vi "Format timestamp into string vs Get Time String.vi"() -> ()   [LabVIEW 2020]
panel:
  out "concatenated string 2":string
  out "concatenated string":string
  out "unit (ms) 2":dbl[](graph)
  out "inside 2":i32
  out "outside 2":i32
  out "inside":i32
  out "outside":i32
  out "unit (ms)":dbl[][](graph)
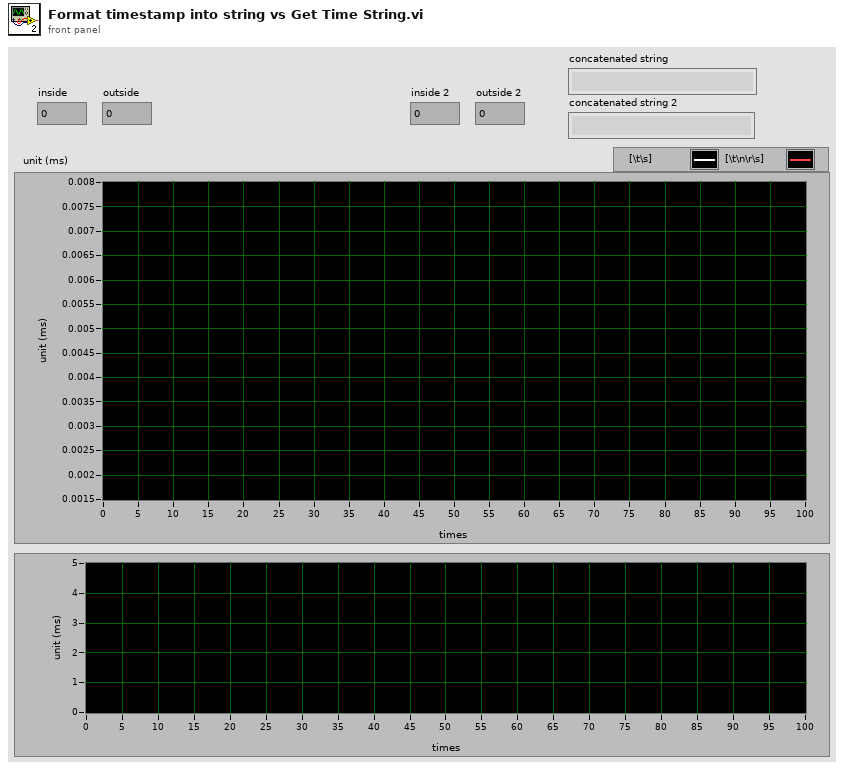
[diagram p1: front panel]
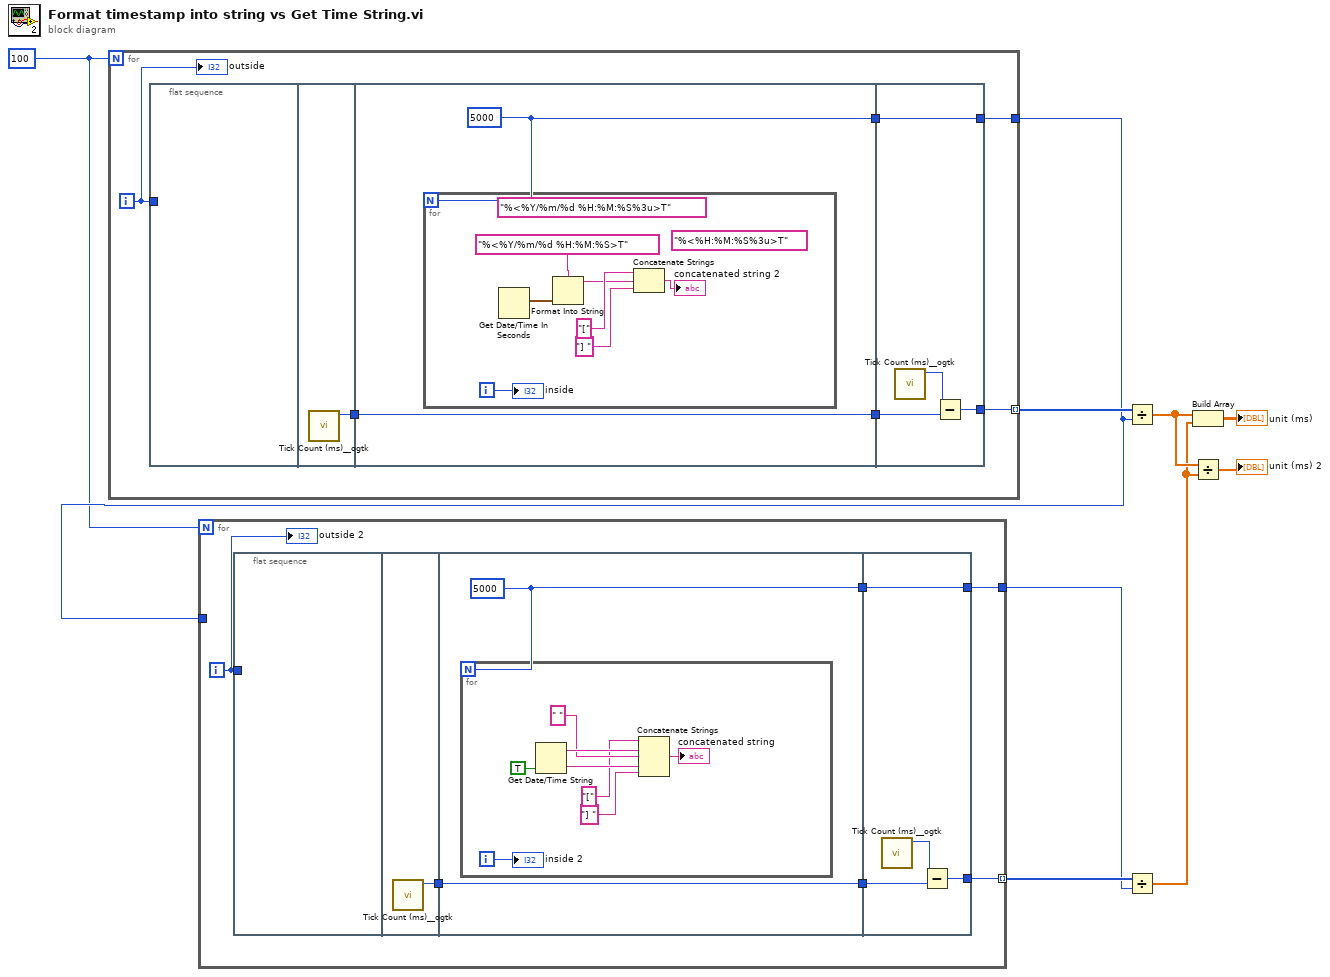
[diagram p0: block diagram]
diagram:
  w4 = 100
  n1 = for {
    N: w4 -> [_]
    tunnel: [w13] -> w9 mode=indexing
    tunnel: [w12] -> w5
    i -> [w10]
    n2 = flat-sequence {
      tunnel: w10 -> [_]
      tunnel: [w16] -> w15
      tunnel: w15 -> [w18]
      tunnel: [w18] -> w14
      tunnel: [w17] -> w11
      tunnel: w14 -> [w28]
      tunnel: [w27] -> w13
      tunnel: [w26] -> w12
      tunnel: w11 -> [w26]
      frame #0 {
      }
      frame #1 {
        n3 = call <userlib>:"Tick Count (ms)__ogtk.vi"() -> ("millisecond timer value"=w16:u32)  [unwired: 10 in, 1 out]
      }
      frame #2 {
        w17 = 5000
        n4 = for {
          N: w17 -> [_]
          i -> [w25]
          (unwired) "%<%H:%M:%S%3u>T" ("format string")
          (unwired) "%<%Y/%m/%d %H:%M:%S%3u>T" ("format string")
          n5 = Get Date/Time In Seconds() -> (seconds since 1Jan1904=w22:timestamp)
          n6 = Format Into String(format string="%<%Y/%m/%d %H:%M:%S>T", w22) -> (resulting string=w21:string)  [unwired: 2 in, 1 out]
          n7 = Concatenate Strings("[" ("string"), w21, "] " ("string")) -> (→"concatenated string 2":string)
          "inside" <- w25
        }
      }
      frame #3 {
        n8 = call <userlib>:"Tick Count (ms)__ogtk.vi"() -> ("millisecond timer value"=w29:u32)  [unwired: 10 in, 1 out]
        n9 = Subtract(x=w29, y=w28) -> (x-y=w27:u32)
      }
    }
    "outside" <- w10
  }
  n10 = for {
    N: w4 -> [_]
    tunnel: [w33] -> w7 mode=indexing
    tunnel: [w32] -> w6
    tunnel: w5 -> [_]
    i -> [w30]
    n11 = flat-sequence {
      tunnel: w30 -> [_]
      tunnel: [w36] -> w35
      tunnel: w35 -> [w38]
      tunnel: [w38] -> w34
      tunnel: [w37] -> w31
      tunnel: w34 -> [w49]
      tunnel: [w48] -> w33
      tunnel: [w47] -> w32
      tunnel: w31 -> [w47]
      frame #0 {
      }
      frame #1 {
        n12 = call <userlib>:"Tick Count (ms)__ogtk.vi"() -> ("millisecond timer value"=w36:u32)  [unwired: 10 in, 1 out]
      }
      frame #2 {
        w37 = 5000
        n13 = for {
          N: w37 -> [_]
          i -> [w46]
          n14 = Get Date/Time String(want seconds? (F)=TRUE) -> (date string=w44:string, time string=w43:string)  [unwired: 2 in]
          n15 = Concatenate Strings("[" ("string"), w44, " " ("string"), w43, "] " ("string")) -> (→"concatenated string":string)
          "inside 2" <- w46
        }
      }
      frame #3 {
        n16 = call <userlib>:"Tick Count (ms)__ogtk.vi"() -> ("millisecond timer value"=w50:u32)  [unwired: 10 in, 1 out]
        n17 = Subtract(x=w50, y=w49) -> (x-y=w48:u32)
      }
    }
    "outside 2" <- w30
  }
  n18 = Divide(x=w9, y=w5) -> (x/y=w2:dbl[])
  n19 = Divide(x=w7, y=w6) -> (x/y=w1:dbl[])
  n20 = Build Array(w2, w1) -> (→"unit (ms)":dbl[][])
  n21 = Divide(x=w2, y=w1) -> (x/y=→"unit (ms) 2":dbl[])
